vi "OFDM_Modulation.vi"(11 "Input sequence":cdb[](array[numeric])) -> (3 "Output sequence":cdb[](array[numeric]))   [LabVIEW 2022 SP3]
uses:
  <vilib>/Analysis/2dsp.llb/Inverse Complex FFT.vi
  <vilib>/Analysis/NI_AALPro.lvlib
panel:
  out "size(s)":i32
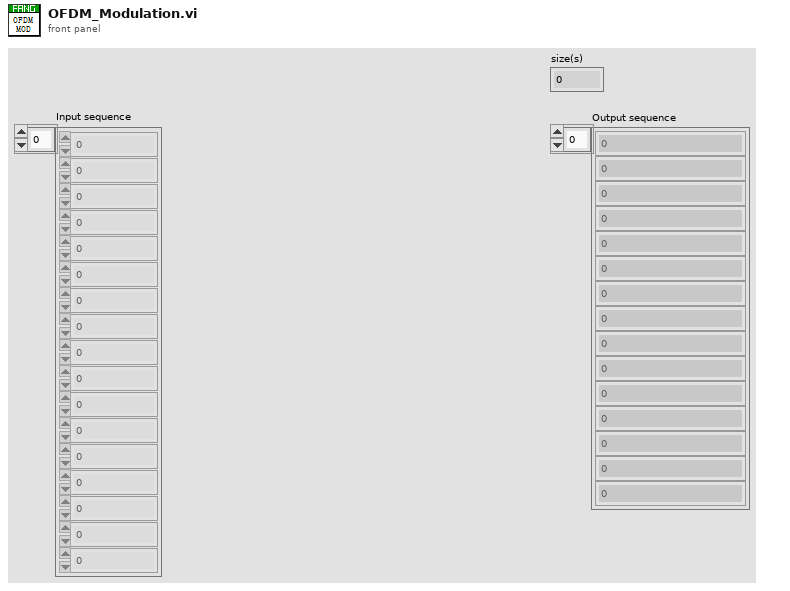
[diagram p1: front panel]
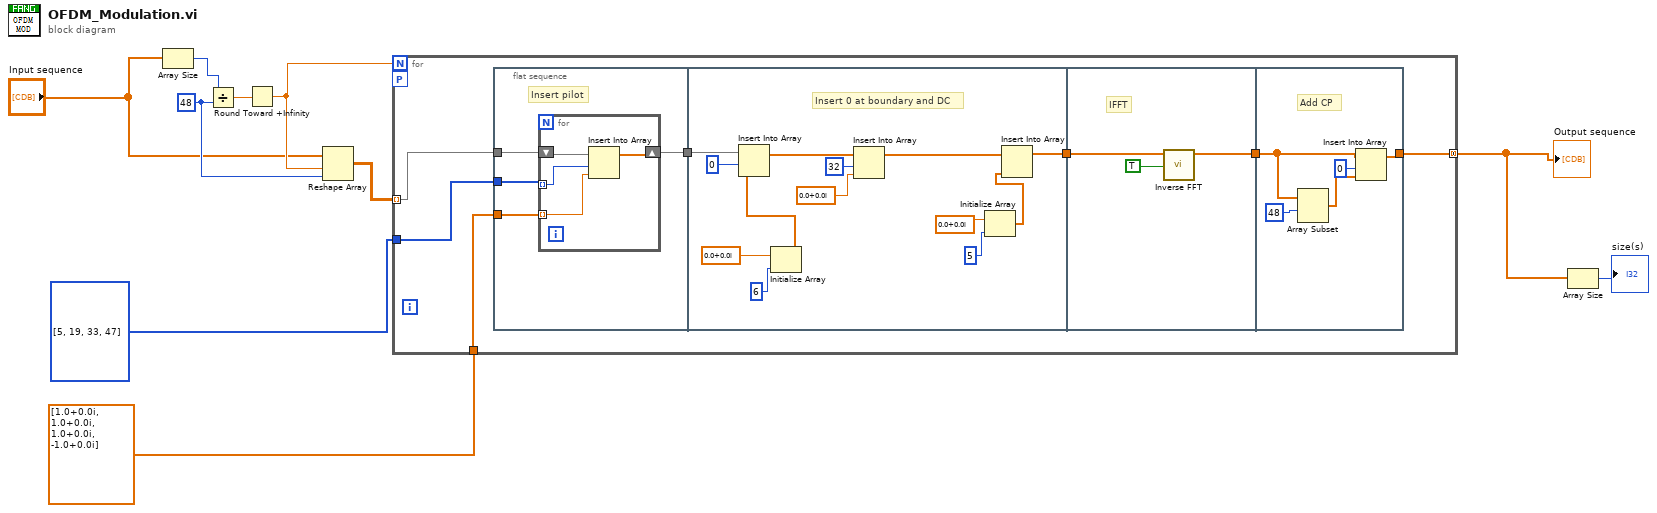
[diagram p0: block diagram]
diagram:
  w6 = 48 ("y")
  n1 = Array Size(array="Input sequence") -> (size(s)=w10:i32)
  n2 = Divide(x=w10, y=w6) -> (x/y=w9:dbl)
  n3 = Round Toward +Infinity(x=w9) -> (ceil(x): smallest int >= x=w7:dbl)
  n4 = Reshape Array("Input sequence", w7, w6) -> (w8:cdb[][])
  n5 = for {
    N: w7 -> [_]
    tunnel: w8 -> [w17] mode=indexing
    tunnel: i32[] [5, 19, 33, 47] -> [w16]
    tunnel: [w13] -> w4 mode=concatenating
    tunnel: cdb[] [1.0+0.0i, 1.0+0.0i, 1.0+0.0i, -1.0+0.0i] -> [w11]
    workers-P: _ -> [_]
    n6 = flat-sequence {
      tunnel: w17 -> [w20]
      tunnel: w16 -> [w21]
      tunnel: [w19] -> w15
      tunnel: w11 -> [w18]
      tunnel: w15 -> [w38]
      tunnel: [w30] -> w14
      tunnel: w14 -> [w41]
      tunnel: [w39] -> w12
      tunnel: [w42] -> w13
      tunnel: w12 -> [w45]
      frame #0 {
        # "Insert pilot"
        n7 = for {
          tunnel: w21 -> [w25] mode=indexing
          shift-right: [w23] -> w19
          shift-left: w20 -> [w24]
          tunnel: w18 -> [w22] mode=indexing
          n8 = Insert Into Array(array=w24, index=w25, new element=w22) -> (w23:cdb[])
        }
      }
      frame #1 {
        # "Insert 0 at boundary and DC"
        n9 = Initialize Array(cdb 0.0+0.0i ("element"), 6 ("dimension size")) -> (w35:cdb[])
        n10 = Insert Into Array(array=w38, index=0, new element=w35) -> (w29:cdb[])
        n11 = Insert Into Array(array=w29, index=32, new element=cdb 0.0+0.0i ("element")) -> (w26:cdb[])
        n12 = Initialize Array(cdb 0.0+0.0i ("element"), 5 ("dimension size")) -> (w31:cdb[])
        n13 = Insert Into Array(array=w26, new element=w31) -> (w30:cdb[])  [unwired: 1 in]
      }
      frame #2 {
        # "IFFT"
        n14 = call-poly <vilib>:"Inverse FFT.vi"("shift?"=TRUE, "FFT {X}"=w41) -> ("X"=w39:cdb[])  [unwired: 8 in, 1 out]
      }
      frame #3 {
        # "Add CP"
        n15 = Array Subset(array=w45, index=48) -> (w44:cdb[])  [unwired: 1 in]
        n16 = Insert Into Array(array=w45, index=0, new element=w44) -> (w42:cdb[])
      }
    }
  }
  "Output sequence" <- w4
  n17 = Array Size(array=w4) -> (size(s)=→"size(s)":i32)
